vi "Read Sweep Configuration File.vi"(8 "error in (no error)":errorcluster, 10 "Path":path, 11 "SweepControl in":refnum<class "SweepControl.lvclass">) -> (0 "error out":errorcluster, 2 "Data":variant, 3 "SweepControl out":refnum<class "SweepControl.lvclass">)   [LabVIEW 2016, in "SweepControl.lvclass"]
uses:
  SweepControl.lvclass
  Transport/subVI/Lockin_Vsg Configuration--Cluster.ctl
  Typedefs/Continuous B Sweep Configuration--Cluster.ctl
  Typedefs/Enum - Experiments.ctl
  Control Experiment/Typedefs/Experiment Description--cluster.ctl
  Control Experiment/Typedefs/Instrument--enum.ctl
  Control Experiment/Typedefs/Wiring Description--cluster.ctl
  <userlib>/LevyLab/Lockin-Multichannel/LockinDAQ/Typedefs/AO-cluster.ctl
  <userlib>/LevyLab/Lockin-Multichannel/LockinDAQ/Typedefs/AO_Amp-array.ctl
  <userlib>/LevyLab/Lockin-Multichannel/LockinDAQ/Typedefs/AO_DC-array.ctl
  <userlib>/LevyLab/Lockin-Multichannel/LockinDAQ/Typedefs/AO_f-array.ctl
  <userlib>/LevyLab/Lockin-Multichannel/LockinDAQ/Typedefs/AO_phi-array.ctl
  <userlib>/LevyLab/Lockin-Multichannel/LockinDAQ/Typedefs/Function-array.ctl
  <userlib>/LevyLab/Lockin-Multichannel/LockinDAQ/Typedefs/Function-enum.ctl
  <userlib>/LevyLab/Lockin-Multichannel/LockinDAQ/Typedefs/REF-cluster.ctl
  <userlib>/LevyLab/Lockin-Multichannel/LockinDAQ/Typedefs/REF_f-array.ctl
  <userlib>/LevyLab/Lockin-Multichannel/LockinDAQ/Typedefs/REF_phi-array.ctl
  <userlib>/LevyLab/Krohn Hite 7008/typedefs/KH_control_array.ctl
  <userlib>/LevyLab/Krohn Hite 7008/typedefs/KH_control.ctl
  <userlib>/LevyLab/Krohn Hite 7008/typedefs/Channel-Enum.ctl
  <userlib>/LevyLab/Krohn Hite 7008/typedefs/Gain-Enum.ctl
  <userlib>/LevyLab/Krohn Hite 7008/typedefs/Shunt-Enum.ctl
  <userlib>/LevyLab/Krohn Hite 7008/typedefs/Input Configuration-Enum.ctl
  Typedefs/Sweep Control Configuration--Cluster.ctl
  Typedefs/ScanParamters.ctl
  Typedefs/Cluster - ScanParamters.ctl
  Typedefs/ScanControl.ctl
  Typedefs/Cluster - ScanControl.ctl
  Typedefs/Enum - Priority.ctl
  Typedefs/Enum - Action.ctl
  <vilib>/addons/_JKI.lib/Serialization/JSON/JKI JSON Serialization.lvlib
  Transport/Transport.lvclass
  <userlib>/LevyLab/Krohn Hite 7008/Instrument.KH7008.lvclass
  Control Experiment/Control Experiment.lvclass
  <userlib>/LevyLab/Lockin-Multichannel/LockinDAQ/LockinDAQ.lvclass
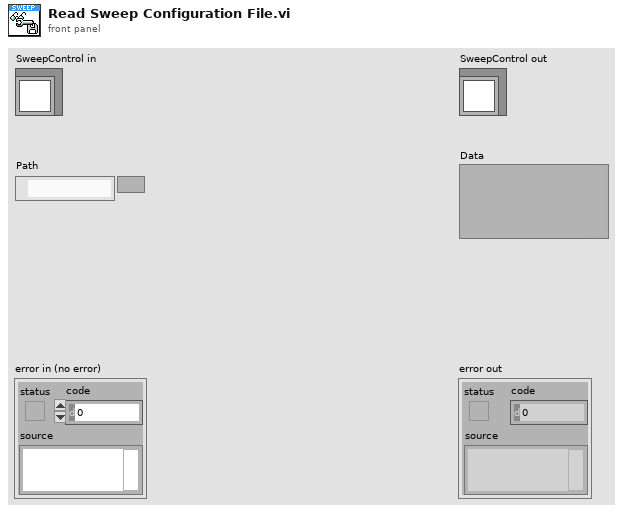
[diagram p1: front panel]
types:
  T1 = typedef "Transport.lvclass/Lockin_Vsg Configuration--Cluster.ctl" = cluster{"Sweep Time (s)":dbl, "Sweep Start (V)":dbl, "Sweep End (V)":dbl, "Sweep Channel":i32}
  T2 = typedef "SweepControl.lvclass/Continuous B Sweep Configuration--Cluster.ctl" = cluster{"Continuous B Sweep":cluster{"Experiment":T3, "B field values":dbl[]}, "Experiment Description":T4, "Wiring Configuration":T6, "Lockin":cluster{"Channels: AO":T7, "Channels: Lockin":T14}, "Krohn Hite":cluster{"Channel Setting":T17}}
  T3 = typedef "SweepControl.lvclass/Enum - Experiments.ctl" = enum16{"IV", "Lockin_time", "Lockin_Vsg", "Lockin (experimental)"}
  T4 = typedef "Control Experiment.lvclass/Experiment Description--cluster.ctl" = cluster{"User":string, "Device":string, "Device Path":path, "Device Description":string, "Experiment Path":path, "Experiment Description":string, "Instrument":T5, "Sweep":cluster{"key":string, "value":variant}[]}
  T5 = typedef "Control Experiment.lvclass/Instrument--enum.ctl" = enum16{"PPMS", "PPMS2", "MFP3D", "CYPHER", "THz1", "THz2", "MNK", "CF900", "JEOL", "AGILENT"}
  T6 = typedef "Control Experiment.lvclass/Wiring Description--cluster.ctl" = cluster{"Lockin Ch":enum16{"1", "2", "3", "4", "5", "6", "7", "8"}[], "KH":cluster{"Electrodes":string[], "Labels":string[]}, "not KH":cluster{"Electrodes":string[], "Labels":string[]}}
  T7 = typedef "LockinDAQ.lvclass/AO-cluster.ctl" = cluster{"AO Amp (V)":T8, "AO DC (V)":T9, "AO f (Hz)":T10, "AO Phase (°)":T11, "Function":T12, "I+":bool[], "Sweeping":bool[]}
  T8 = typedef "LockinDAQ.lvclass/AO_Amp-array.ctl" = dbl[]
  T9 = typedef "LockinDAQ.lvclass/AO_DC-array.ctl" = dbl[]
  T10 = typedef "LockinDAQ.lvclass/AO_f-array.ctl" = dbl[]
  T11 = typedef "LockinDAQ.lvclass/AO_phi-array.ctl" = dbl[]
  T12 = typedef "LockinDAQ.lvclass/Function-array.ctl" = T13[]
  T13 = typedef "LockinDAQ.lvclass/Function-enum.ctl" = enum16{"Sine", "Triangle", "Square", "Sawtooth"}
  T14 = typedef "LockinDAQ.lvclass/REF-cluster.ctl" = cluster{"REF f (Hz)":T15, "REF phi (°)":T16}
  T15 = typedef "LockinDAQ.lvclass/REF_f-array.ctl" = dbl[]
  T16 = typedef "LockinDAQ.lvclass/REF_phi-array.ctl" = dbl[]
  T17 = typedef "Instrument.KH7008.lvclass/KH_control_array.ctl" = T18[]
  T18 = typedef "Instrument.KH7008.lvclass/KH_control.ctl" = cluster{"Channel":T19, "Gain":T20, "Shunt Resistor":T21, "Input Config":T22}
  T19 = typedef "Instrument.KH7008.lvclass/Channel-Enum.ctl" = enum16{"Channel 1", "Channel 2", "Channel 3", "Channel 4", "Channel 5", "Channel 6", "Channel 7", "Channel 8"}
  T20 = typedef "Instrument.KH7008.lvclass/Gain-Enum.ctl" = enum16{"1x", "10x", "100x", "1000x"}
  T21 = typedef "Instrument.KH7008.lvclass/Shunt-Enum.ctl" = enum16{"Open", "50 Ohms", "500 Ohms", "5k Ohms", "50k Ohms"}
  T22 = typedef "Instrument.KH7008.lvclass/Input Configuration-Enum.ctl" = enum16{"Ground", "SE+ (-gnd)", "SE- (+gnd)", "Differential"}
  T23 = typedef "SweepControl.lvclass/Sweep Control Configuration--Cluster.ctl" = cluster{"Sweep Control":cluster{"Experiment":T3, "Scan parameters":T24, "Scan control":T26}, "Experiment Description":T4, "Wiring Configuration":T6, "Lockin":cluster{"Channels: AO":T7, "Channels: Lockin":T14}, "Krohn Hite":cluster{"Channel Setting":T17}}
  T24 = typedef "SweepControl.lvclass/ScanParamters.ctl" = T25[]
  T25 = typedef "SweepControl.lvclass/Cluster - ScanParamters.ctl" = cluster{"Start":dbl, "End":dbl, "Step":dbl, "Rate":dbl, "wait (ms)":u32, "Address":string, "channel":i32}
  T26 = typedef "SweepControl.lvclass/ScanControl.ctl" = T27[]
  T27 = typedef "SweepControl.lvclass/Cluster - ScanControl.ctl" = cluster{"Priority":T28, "Scan name":T29}
  T28 = typedef "SweepControl.lvclass/Enum - Priority.ctl" = enum16{"Priority 0", "Priority 1", "Priority 2", "Priority 3", "Priority 4", "Priority 5"}
  T29 = typedef "SweepControl.lvclass/Enum - Action.ctl" = enum16{"OFF", "DSA_Vamp", "DSA_freq", "DSA_Vsg1", "DSA_Vsg2", "DSA_Vsg3", "DAQ_Vbg", "B_Field", "Humidity", "Temp", "MW_freq1", "MW_freq2", "MW_amplitude1", "MW_amplitude2"}
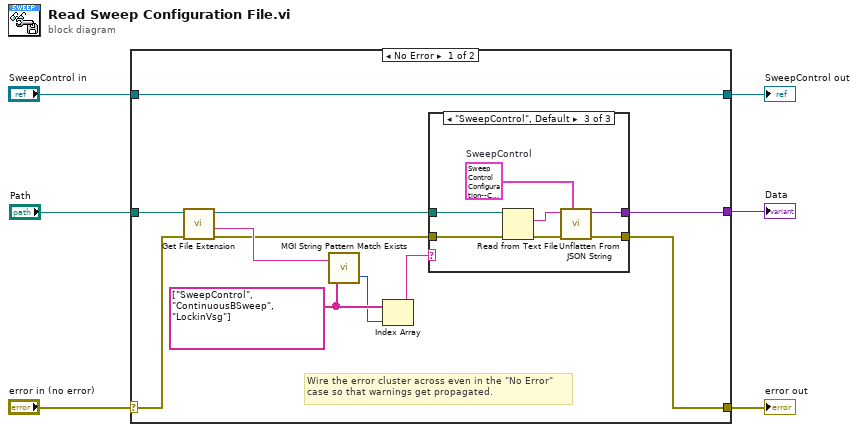
[diagram p0: block diagram]
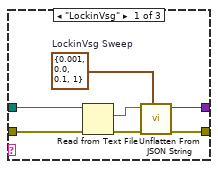
[diagram p2: hidden frame]
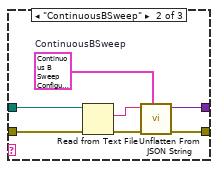
[diagram p3: hidden frame]
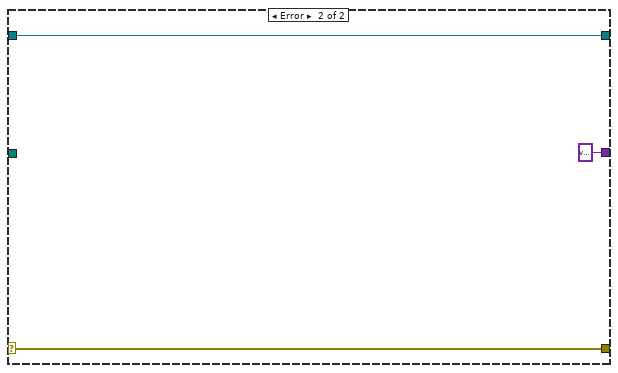
[diagram p4: hidden frame]
diagram:
  n1 = case shown="No Error" "error in (no error)" {
    selector: "error in (no error)" -> [w8 w41]
    tunnel: [w7 w41] -> w5
    tunnel: [w17 w40] -> w3
    tunnel: "SweepControl in" -> [w17 w40]
    tunnel: "Path" -> [w16 _]
    tunnel: [w9 variant ("Variant")] -> w1
    frame No Error {
      w14 = string[] ["SweepControl", "ContinuousBSweep", "LockinVsg"] ("Patterns to Try")
      # "Wire the error cluster across even in the \"No Error\"\ncase so that warnings get propagated."
      n2 = call <vilib>:"Get File Extension.vi"("error in (no error)"=w8, "file"=w16) -> ("error out"=w11:errorcluster, "filename without extension"=w13:string, "dup file"=w10:path)  [unwired: 5 in, 2 out]
      n3 = call <userlib>:"MGI String Pattern Match Exists.vi"("Patterns to Try"=w14, "String"=w13) -> ("Index of First Pattern Matched"=w12:i32)  [unwired: 1 out]
      n4 = Index Array(array=w14, index=w12) -> (element=w15:string)
      n5 = case shown="\"SweepControl\", Default" w15 {
        tunnel: w11 -> [w22 w29 w36]
        tunnel: w10 -> [w21 w28 w35]
        tunnel: [w19 w27 w34] -> w9
        tunnel: [w18 w26 w33] -> w7
        frame "LockinVsg" {
          w20 = T1 {"Sweep Time (s)"=0.001, "Sweep Start (V)"=0.0, "Sweep End (V)"=0.1, "Sweep Channel"=1}  # LockinVsg Sweep
          n6 = Read from Text File(file (use dialog)=w21, error in=w22) -> (text=w23:string, error out=w24:errorcluster)  [unwired: 2 in, 2 out]
          n7 = call <vilib>:"Unflatten From JSON String.vi"("Type and Defaults"=w20, "error in (no error)"=w24, "JSON String"=w23) -> ("error out"=w18:errorcluster, "Variant"=w19:variant)  [unwired: 7 in]
        }
        frame "ContinuousBSweep" {
          w25 = T2 {"Continuous B Sweep"={"Experiment"=enum."IV", "B field values"=[]}, "Experiment Description"={"User"="", "Device"="", "Device Path"=path "", "Device Description"="", "Experiment Path"=path "", "Experiment Description"="", "Instrument"=enum."MNK", "Sweep"=[{"key"="OFF", "value"=variant}, {"key"="OFF", "value"=variant}, {"key"="OFF", "value"=variant}, {"key"="OFF", "value"=variant}]}, "Wiring Configuration"={"Lockin Ch"=[], "KH"={"Electrodes"=[], "Labels"=[]}, "not KH"={"Electrodes"=[], "Labels"=[]}}, "Lockin"={"Channels: AO"={"AO Amp (V)"=[0.01, 0.0, 0.0, 0.0, 0.0, 0.0, 0.0, 0.0], "AO DC (V)"=[0.0, 0.0, 0.0, 0.0, 0.0, 0.0, 0.0, 0.0], "AO f (Hz)"=[13.1, 13.0, 13.0, 13.0, 13.0, 13.0, 13.0, 13.0], "AO Phase (°)"=[0.0, 0.0, 0.0, 0.0, 0.0, 0.0, 0.0, 0.0], "Function"=[enum."Sine", enum."Sine", enum."Sine", enum."Sine", enum."Sine", enum."Sine", enum."Sine", enum."Sine"], "I+"=[], "Sweeping"=[]}, "Channels: Lockin"={"REF f (Hz)"=[13.0], "REF phi (°)"=[0.0, 0.0, 0.0, 0.0, 0.0, 0.0, 0.0, 0.0]}}, "Krohn Hite"={"Channel Setting"=[]}}  # ContinuousBSweep
          n8 = Read from Text File(file (use dialog)=w28, error in=w29) -> (text=w30:string, error out=w31:errorcluster)  [unwired: 2 in, 2 out]
          n9 = call <vilib>:"Unflatten From JSON String.vi"("Type and Defaults"=w25, "error in (no error)"=w31, "JSON String"=w30) -> ("error out"=w26:errorcluster, "Variant"=w27:variant)  [unwired: 7 in]
        }
        frame "SweepControl", Default {
          w32 = T23 {"Sweep Control"={"Experiment"=enum."IV", "Scan parameters"=[], "Scan control"=[]}, "Experiment Description"={"User"="", "Device"="", "Device Path"=path "", "Device Description"="", "Experiment Path"=path "", "Experiment Description"="", "Instrument"=enum."MNK", "Sweep"=[{"key"="OFF", "value"=variant}, {"key"="OFF", "value"=variant}, {"key"="OFF", "value"=variant}, {"key"="OFF", "value"=variant}]}, "Wiring Configuration"={"Lockin Ch"=[], "KH"={"Electrodes"=[], "Labels"=[]}, "not KH"={"Electrodes"=[], "Labels"=[]}}, "Lockin"={"Channels: AO"={"AO Amp (V)"=[0.01, 0.0, 0.0, 0.0, 0.0, 0.0, 0.0, 0.0], "AO DC (V)"=[0.0, 0.0, 0.0, 0.0, 0.0, 0.0, 0.0, 0.0], "AO f (Hz)"=[13.1, 13.0, 13.0, 13.0, 13.0, 13.0, 13.0, 13.0], "AO Phase (°)"=[0.0, 0.0, 0.0, 0.0, 0.0, 0.0, 0.0, 0.0], "Function"=[enum."Sine", enum."Sine", enum."Sine", enum."Sine", enum."Sine", enum."Sine", enum."Sine", enum."Sine"], "I+"=[], "Sweeping"=[]}, "Channels: Lockin"={"REF f (Hz)"=[13.0], "REF phi (°)"=[0.0, 0.0, 0.0, 0.0, 0.0, 0.0, 0.0, 0.0]}}, "Krohn Hite"={"Channel Setting"=[]}}  # SweepControl
          n10 = Read from Text File(file (use dialog)=w35, error in=w36) -> (text=w37:string, error out=w38:errorcluster)  [unwired: 2 in, 2 out]
          n11 = call <vilib>:"Unflatten From JSON String.vi"("Type and Defaults"=w32, "error in (no error)"=w38, "JSON String"=w37) -> ("error out"=w33:errorcluster, "Variant"=w34:variant)  [unwired: 7 in]
        }
      }
    }
    frame Error {
    }
  }
  "error out" <- w5
  "SweepControl out" <- w3
  "Data" <- w1
